vi "SetDefaultPort.vi"(8 "error in (no error)":errorcluster, 9 "IP Address":string, 10 "Port":u16, 11 "Config in":T1) -> (0 "error out":errorcluster, 3 "Config out":T1)   [LabVIEW 2016]
uses:
  <vilib>/WebServerConfig/Config.ctl
  <vilib>/WebServerConfig/Server.ctl
  <vilib>/WebServerConfig/Alias.ctl
  <vilib>/WebServerConfig/ErrorDocument.ctl
  <vilib>/WebServerConfig/Action.ctl
  <vilib>/WebServerConfig/Redirect.ctl
  <vilib>/WebServerConfig/Interface.ctl
  <vilib>/WebServerConfig/AddHandler.ctl
  <vilib>/WebServerConfig/SSL.ctl
  <vilib>/WebServerConfig/CustomLog.ctl
  <vilib>/WebServerConfig/LoadModule.ctl
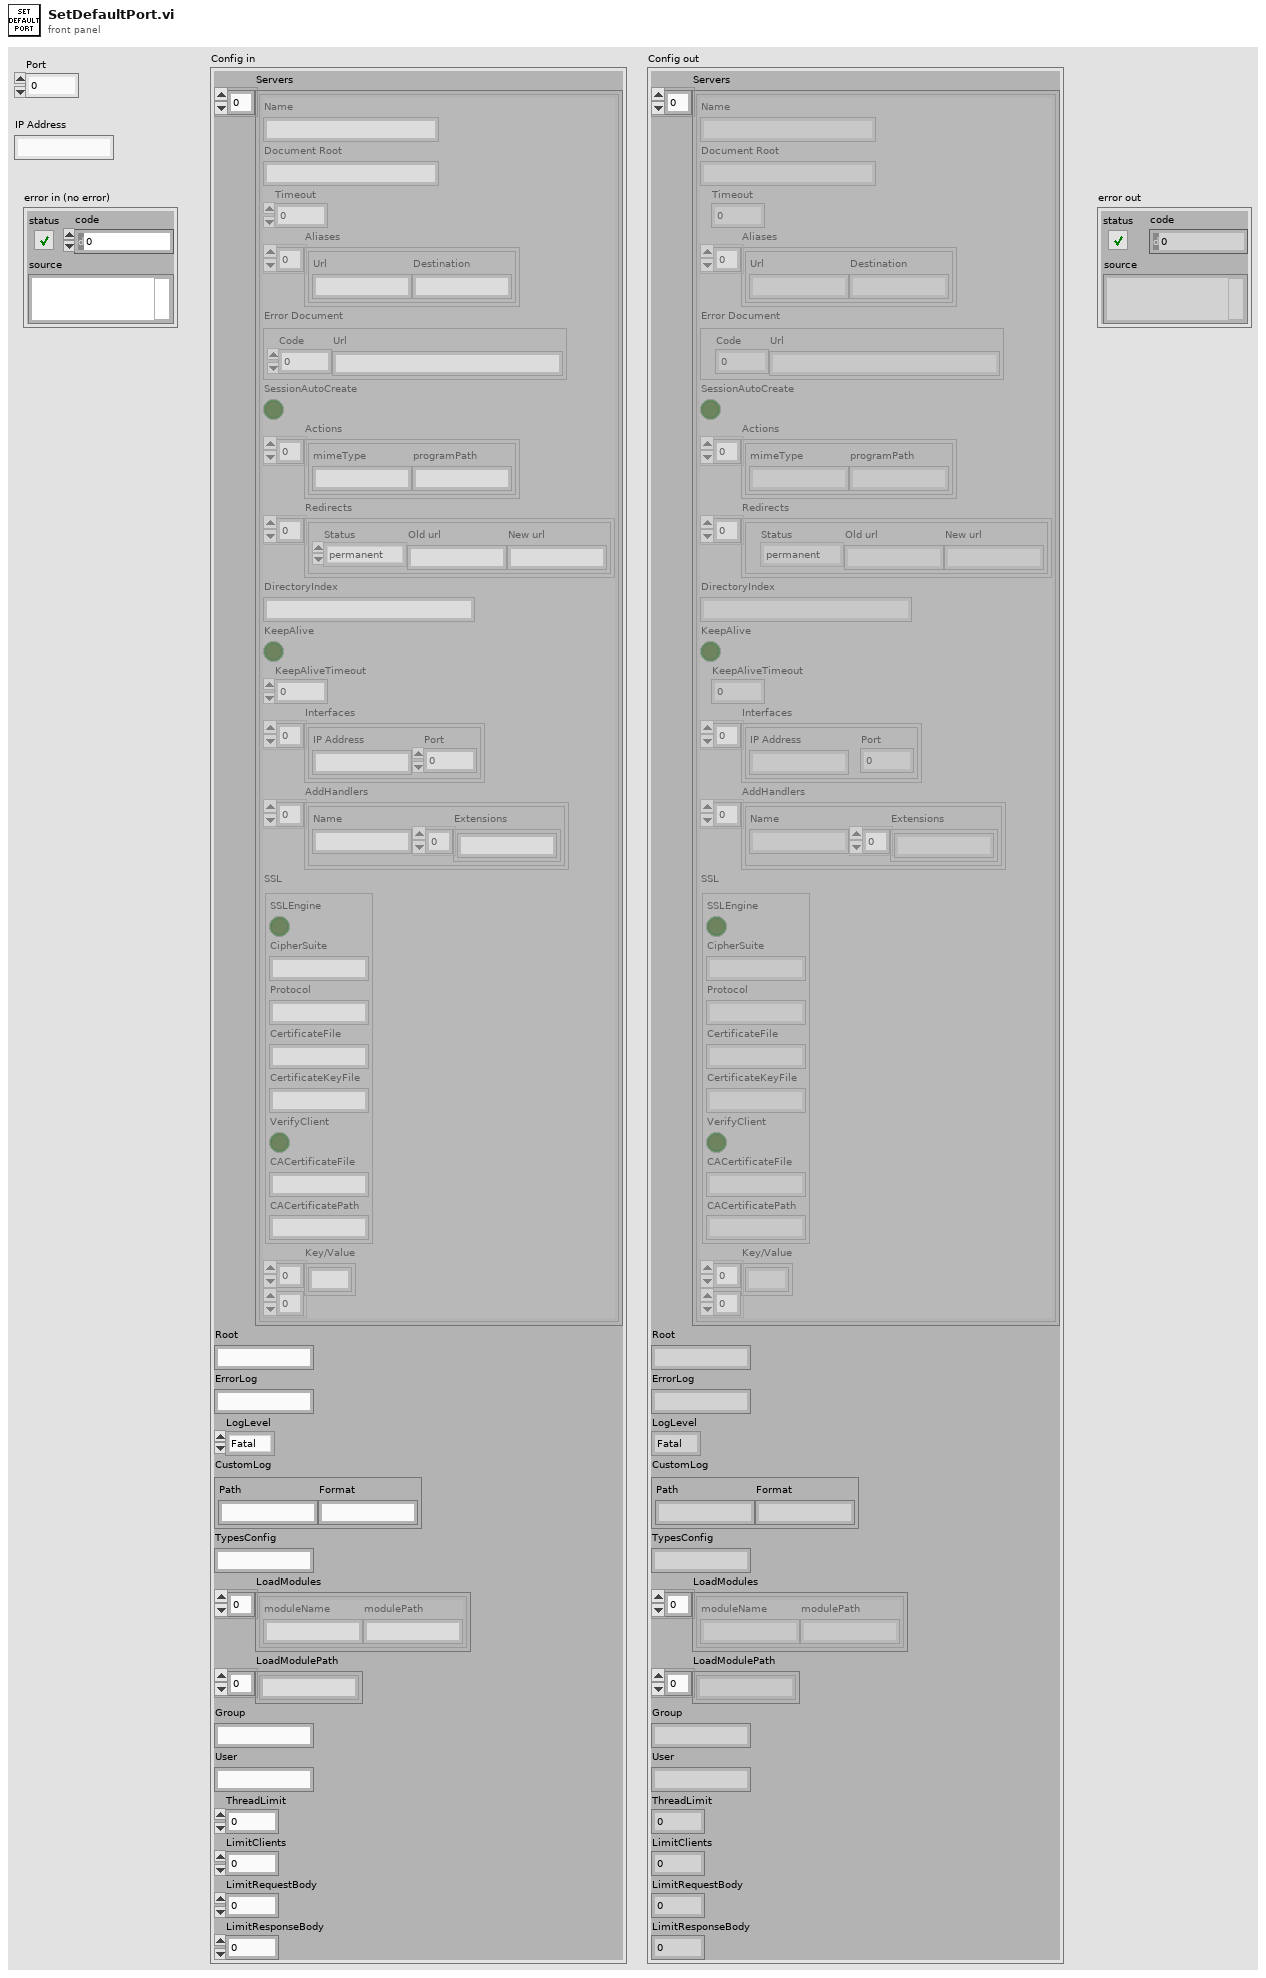
[diagram p1: front panel]
types:
  T1 = typedef "Config.ctl" = cluster{"Servers":T2[], "Root":string, "ErrorLog":string, "LogLevel":enum16{"Fatal", "Error", "Warn", "Info", "Debug", "5", "6", "7", "8", "Verbose"}, "CustomLog":T10, "TypesConfig":string, "LoadModules":T11[], "LoadModulePath":string[], "Group":string, "User":string, "ThreadLimit":u32, "LimitClients":u32, "LimitRequestBody":u32, "LimitResponseBody":u32}
  T2 = typedef "Server.ctl" = cluster{"Name":string, "Document Root":string, "Timeout":u32, "Aliases":T3[], "Error Document":T4, "SessionAutoCreate":bool, "Actions":T5[], "Redirects":T6[], "DirectoryIndex":string, "KeepAlive":bool, "KeepAliveTimeout":u32, "Interfaces":T7[], "AddHandlers":T8[], "SSL":T9, "Key/Value":string[][]}
  T3 = typedef "Alias.ctl" = cluster{"Url":string, "Destination":string}
  T4 = typedef "ErrorDocument.ctl" = cluster{"Code":u16, "Url":string}
  T5 = typedef "Action.ctl" = cluster{"mimeType":string, "programPath":string}
  T6 = typedef "Redirect.ctl" = cluster{"Status":enum16{"permanent", "temp", "seeother", "gone"}, "Old url":string, "New url":string}
  T7 = typedef "Interface.ctl" = cluster{"IP Address":string, "Port":u16}
  T8 = typedef "AddHandler.ctl" = cluster{"Name":string, "Extensions":string[]}
  T9 = typedef "SSL.ctl" = cluster{"SSLEngine":bool, "CipherSuite":string, "Protocol":string, "CertificateFile":string, "CertificateKeyFile":string, "VerifyClient":bool, "CACertificateFile":string, "CACertificatePath":string}
  T10 = typedef "CustomLog.ctl" = cluster{"Path":string, "Format":string}
  T11 = typedef "LoadModule.ctl" = cluster{"moduleName":string, "modulePath":string}
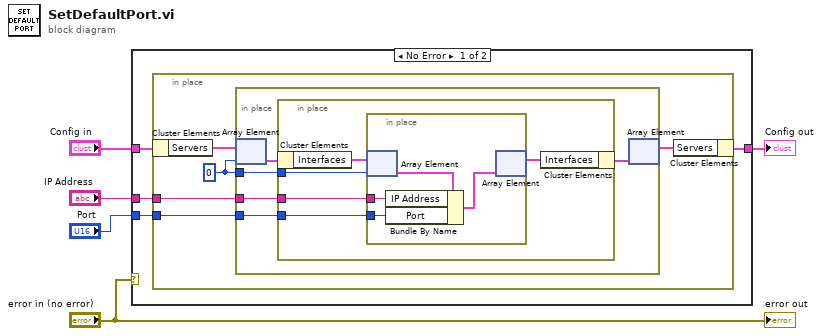
[diagram p0: block diagram]
diagram:
  n1 = case shown="No Error" "error in (no error)" {
    tunnel: "Config in" -> [w9 w29]
    tunnel: [w8 w29] -> w3
    tunnel: "Port" -> [w7 _]
    tunnel: "IP Address" -> [w6 _]
    frame No Error {
      n2 = in-place {
        in-place-border: w7 -> [w11]
        in-place-border: w6 -> [w10]
        w13 = 0
        n3 = in-place-cluster #1(w9) -> ("Servers"=w14:T2[])
        n4 = in-place {
          in-place-border: w13 -> [w17]
          in-place-border: w11 -> [w16]
          in-place-border: w10 -> [w15]
          n5 = in-place-array #2(w14, w13) -> (w19:T2)
          n6 = in-place {
            in-place-border: w17 -> [w23]
            in-place-border: w16 -> [w21]
            in-place-border: w15 -> [w20]
            n7 = in-place-cluster #3(w19) -> ("Interfaces"=w24:T7[])
            n8 = in-place {
              in-place-border: w21 -> [w26]
              in-place-border: w20 -> [w25]
              n9 = in-place-array #4(w24, w23) -> (w28:T7)
              n10 = Bundle By Name(cluster=w28, "IP Address"=w25, "Port"=w26) -> (w27:T7)
              n11 = in-place-array #4(w27) -> (w22:T7[])  [unwired: 1 out]
            }
            n12 = in-place-cluster #3("Interfaces"=w22) -> (w18:T2)
          }
          n13 = in-place-array #2(w18) -> (w12:T2[])  [unwired: 1 out]
        }
        n14 = in-place-cluster #1("Servers"=w12) -> (w8:T1)
      }
    }
    frame Error {
    }
  }
  "Config out" <- w3
  "error out" <- "error in (no error)"
